vi "Set Output.vi"(8 "error in (no error)":errorcluster, 10 "Output Voltage [V]":dbl, 11 "Ramp Use Case in":refnum<class "Ramp Voltage.lvclass">) -> (0 "error out":errorcluster, 3 "Ramp Use Case out":refnum<class "Ramp Voltage.lvclass">)   [LabVIEW 2020, in "High Level PSU With Tests.lvlib" / "Ramp Voltage.lvclass"]
uses:
  Ramp Voltage.lvclass
  Ramp Voltage.lvclass/Ramp Voltage.ctl
  Voltage Output/Voltage Output.lvclass
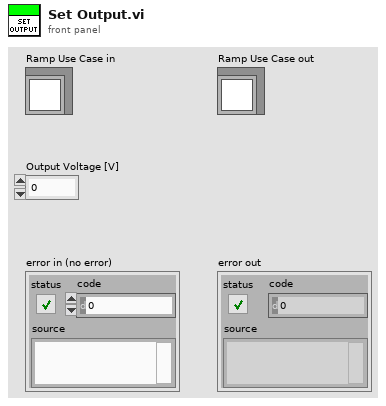
[diagram p1: front panel]
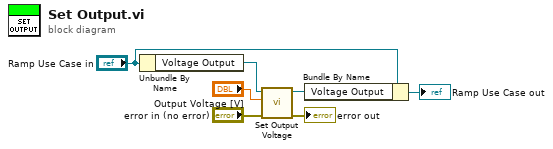
[diagram p0: block diagram]
diagram:
  n1 = Unbundle By Name("Ramp Use Case in") -> ("Voltage Output"=w3:refnum<class "Voltage Output.lvclass">)
  n2 = call-dynamic "Set Output Voltage.vi"("error in (no error)"="error in (no error)", "Voltage [V]"="Output Voltage [V]", "Voltage Output In"=w3) -> ("error out"=→"error out":errorcluster, "Voltage Output Out"=w7:refnum<class "Voltage Output.lvclass">)  [unwired: 7 in]
  n3 = Bundle By Name(cluster="Ramp Use Case in", "Voltage Output"=w7) -> (→"Ramp Use Case out":refnum<class "Ramp Voltage.lvclass">)
